vi "combosToRanges.vi"(11 "combosIn":T1[][](array[typedef]) {"mDot" format="%_4g"; "Setpoint" format="%.2g"; "MFCcapability"."MaxMdot" format="%_4g"; "MFCcapability"."MinMdot" format="%_4g"}) -> (1 "OverallMinMdot(g/min)":dbl, 2 "OverallMaxMdot(g/min)":dbl, 3 "rangesOut":T3[](array[typedef]))   [LabVIEW 2021]
uses:
  ComboRange.ctl
  MFCdescription.ctl
  MFCcapability.ctl
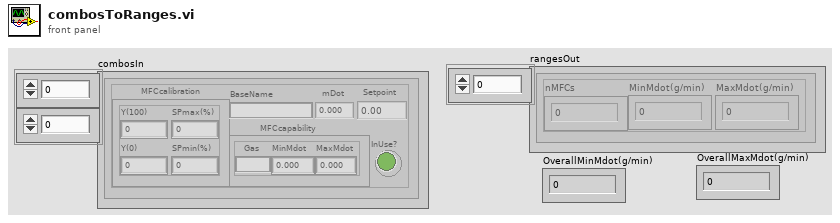
[diagram p1: front panel]
types:
  T1 = typedef "MFCdescription.ctl" = cluster{"BaseName":string, "MFCcalibration":cluster{"Y(100)":dbl, "Y(0)":dbl, "SPmin(%)":dbl, "SPmax(%)":dbl}, "MFCcapability":T2, "InUse?":bool, "Setpoint":dbl, "mDot":dbl}
  T2 = typedef "MFCcapability.ctl" = cluster{"Gas":string, "MinMdot":dbl, "MaxMdot":dbl}
  T3 = typedef "ComboRange.ctl" = cluster{"nMFCs":i32, "MinMdot(g/min)":dbl, "MaxMdot(g/min)":dbl}
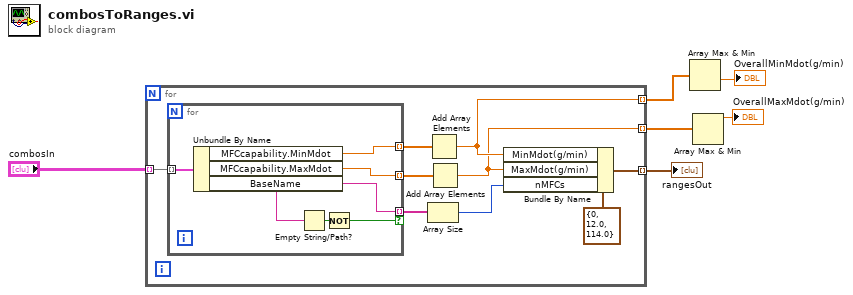
[diagram p0: block diagram]
diagram:
  n1 = for {
    tunnel: "combosIn" -> [w13] mode=indexing
    tunnel: [w9] -> w6 mode=indexing
    tunnel: [w8] -> w4 mode=indexing
    tunnel: [w7] -> w3 mode=indexing
    n2 = for {
      tunnel: [w20] -> w15 mode=indexing
      tunnel: [w19] -> w14 mode=indexing if=w16
      tunnel: w13 -> [w18] mode=indexing
      tunnel: [w17] -> w12 mode=indexing
      n3 = Unbundle By Name(w18) -> ("MFCcapability.MinMdot"=w17:dbl, "MFCcapability.MaxMdot"=w20:dbl, "BaseName"=w19:string)
      n4 = Empty String/Path?(string/path=w19) -> (empty?=w21:bool)
      n5 = Not(x=w21) -> (.not. x?=w16:bool)
    }
    n6 = Array Size(array=w14) -> (size(s)=w10:i32)
    n7 = Add Array Elements(numeric array=w12) -> (sum=w8:dbl)
    n8 = Add Array Elements(numeric array=w15) -> (sum=w7:dbl)
    n9 = Bundle By Name(cluster=T3 {"nMFCs"=0, "MinMdot(g/min)"=12.0, "MaxMdot(g/min)"=114.0} ("Cluster"), "MinMdot(g/min)"=w8, "MaxMdot(g/min)"=w7, "nMFCs"=w10) -> (w9:T3)
  }
  "rangesOut" <- w6
  n10 = Array Max & Min(array=w4) -> (min value=→"OverallMinMdot(g/min)":dbl)  [unwired: 3 out]
  n11 = Array Max & Min(array=w3) -> (max value=→"OverallMaxMdot(g/min)":dbl)  [unwired: 3 out]
